vi "Default Configuration.vi"() -> (1 "Filter order":u32(ring)=1 items=["Order2"=1, "Order4"=3], 2 "Filter frequency":u32(ring) items=["1st Frequency", "2nd Frequency", "3rd Frequency", "4th Frequency", "5th Frequency", "6th Frequency"], 3 "Filter response":u32(ring) items=["Comb"=0, "Butterworth"=2], 4 "channel settings":T1, 5 "Data rate":u32(ring) items=["50.000 kS/s"=0, "33.333 kS/s"=1, "25.000 kS/s"=2, "20.000 kS/s"=3, "16.667 kS/s"=4, "14.286 kS/s"=5, "12.500 kS/s"=6, "11.111 kS/s"=7, "10.000 kS/s"=8, "8.333 kS/s"=9, "7.143 kS/s"=10, "6.250 kS/s"=11, "5.556 kS/s"=12, "5.000 kS/s"=13, "4.545 kS/s"=14, "4.167 kS/s"=15, "3.571 kS/s"=16, "3.125 kS/s"=17, "2.778 kS/s"=18, "2.500 kS/s"=19, "2.273 kS/s"=20, "2.083 kS/s"=21, "2.000 kS/s"=22, "1.786 kS/s"=23, "1.563 kS/s"=24, "1.389 kS/s"=25, "1.250 kS/s"=26, "1.136 kS/s"=27, "1.042 kS/s"=28, "1.000 kS/s"=29, "892.86 S/s"=30, "781.25 S/s"=31, "694.44 S/s"=32, "625.00 S/s"=33, "568.18 S/s"=34, "520.83 S/s"=35, "500.00 S/s"=36, "446.43 S/s"=37, "400.00 S/s"=38, "390.63 S/s"=39, "347.22 S/s"=40, "312.50 S/s"=41, "284.09 S/s"=42, "260.42 S/s"=43, "250.00 S/s"=44, "223.21 S/s"=45, "200.00 S/s"=46, "195.31 S/s"=47, "142.05 S/s"=48, "125.00 S/s"=49, "100.00 S/s"=50, "97.66 S/s"=51, "60.02 S/s"=52, "50.00 S/s"=54, "10.00 S/s"=56], 7 "Field-side power fault detection enable":bool)   [LabVIEW 2020, in "Modules.lvlib" / "9253.lvclass"]
uses:
  9253.lvclass
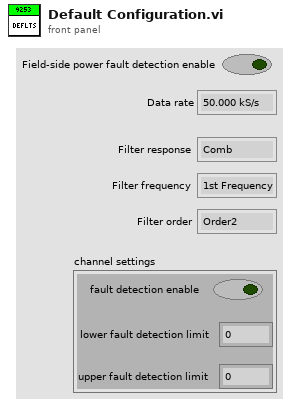
[diagram p1: front panel]
types:
  T1 = cluster{"fault detection enable":bool, "lower fault detection limit":dbl, "upper fault detection limit":dbl}
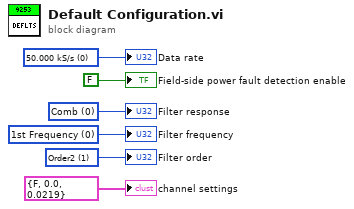
[diagram p0: block diagram]
diagram:
  w6 = u32 0 items=["Comb"=0, "Butterworth"=2] ("Filter response")
  w5 = u32 1 items=["Order2"=1, "Order4"=3] ("Filter order")
  w4 = u32 0 items=["1st Frequency", "2nd Frequency", "3rd Frequency", "4th Frequency", "5th Frequency", "6th Frequency"] ("Filter frequency")
  w3 = u32 0 items=["50.000 kS/s"=0, "33.333 kS/s"=1, "25.000 kS/s"=2, "20.000 kS/s"=3, "16.667 kS/s"=4, "14.286 kS/s"=5, "12.500 kS/s"=6, "11.111 kS/s"=7, "10.000 kS/s"=8, "8.333 kS/s"=9, "7.143 kS/s"=10, "6.250 kS/s"=11, "5.556 kS/s"=12, "5.000 kS/s"=13, "4.545 kS/s"=14, "4.167 kS/s"=15, "3.571 kS/s"=16, "3.125 kS/s"=17, "2.778 kS/s"=18, "2.500 kS/s"=19, "2.273 kS/s"=20, "2.083 kS/s"=21, "2.000 kS/s"=22, "1.786 kS/s"=23, "1.563 kS/s"=24, "1.389 kS/s"=25, "1.250 kS/s"=26, "1.136 kS/s"=27, "1.042 kS/s"=28, "1.000 kS/s"=29, "892.86 S/s"=30, "781.25 S/s"=31, "694.44 S/s"=32, "625.00 S/s"=33, "568.18 S/s"=34, "520.83 S/s"=35, "500.00 S/s"=36, "446.43 S/s"=37, "400.00 S/s"=38, "390.63 S/s"=39, "347.22 S/s"=40, "312.50 S/s"=41, "284.09 S/s"=42, "260.42 S/s"=43, "250.00 S/s"=44, "223.21 S/s"=45, "200.00 S/s"=46, "195.31 S/s"=47, "142.05 S/s"=48, "125.00 S/s"=49, "100.00 S/s"=50, "97.66 S/s"=51, "60.02 S/s"=52, "50.00 S/s"=54, "10.00 S/s"=56] ("Data rate")
  "Filter response" <- w6
  "Filter order" <- w5
  "Filter frequency" <- w4
  "Data rate" <- w3
  "Field-side power fault detection enable" <- FALSE ("Field-side power fault detection enable")
  "channel settings" <- T1 {"fault detection enable"=FALSE, "lower fault detection limit"=0.0, "upper fault detection limit"=0.0219} ("channel settings")
